vi "ObtainQueue.vi"(0 "Queue Name":string, 1 "max queue size (-1, unlimited)":i32, 11 "error in (no error)":errorcluster) -> (4 "MessageQueue":refnum<queue>, 15 "error out":errorcluster)   [LabVIEW 2018, in "ScopePlugins.lvlib"]
uses:
  ScopePlugins.lvlib
  clMessage.ctl
panel:
  # "This obtaind a queue and\nenqueues the \"Initialize\"\nMessage"
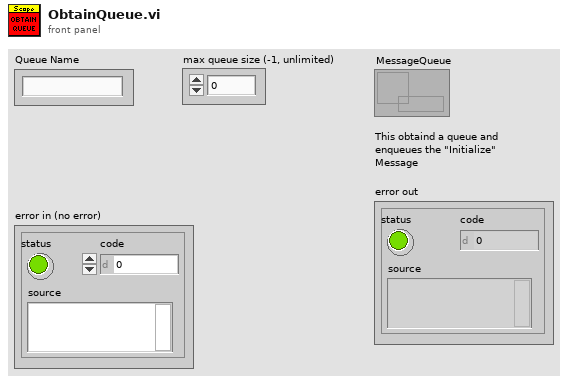
[diagram p1: front panel]
types:
  T1 = typedef "ScopePlugins.lvlib/clMessage.ctl" = cluster{"Message":string, "Message Data":variant}
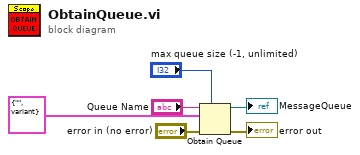
[diagram p0: block diagram]
diagram:
  n1 = Obtain Queue(max queue size (-1, unlimited)="max queue size (-1, unlimited)", name (unnamed)="Queue Name", element data type=T1 {"Message"="", "Message Data"=variant} ("clMessage"), error in (no error)="error in (no error)") -> (queue out=→"MessageQueue":refnum<queue>, error out=→"error out":errorcluster)  [unwired: 1 in, 1 out]
